vi "NMR T2 CPMG Sequence - Large Magnet - PN HPA - 2nd Setup.vi"() -> ()   [LabVIEW 2024]
uses:
  <instrlib>/niFgen/niFgen.llb/niFgen Output Mode.ctl
  <instrlib>/niFgen/niFgen.llb/niFgen Waveform Type.ctl
  <instrlib>/niFgen/niFgen.llb/niFgen_ctl Trigger DigEdge - Edge Values (Ring).ctl
  <instrlib>/niFgen/niFgen.llb/niFgen_ctl Trigger Source Values (Ring).ctl
  <instrlib>/niFgen/niFgen.llb/niFgen Trigger Mode.ctl
  <instrlib>/niScope/Controls/niScope acquisition type.ctl
  <instrlib>/niScope/Controls/niScope trigger slope.ctl
  <instrlib>/niScope/Controls/niScope trigger source.ctl
  <vilib>/Analysis/2dsp.llb/Integral Method.ctl
  <vilib>/Analysis/8numeric.llb/1D Numeric Integration.vi
  <vilib>/Utility/file.llb/Read Delimited Spreadsheet (DBL).vi
  <instrlib>/niFgen/niFgen.llb/niFgen Create Waveform (DBL).vi
  <instrlib>/niScope/Configure/Trigger/niScope Configure Trigger Edge.vi
  <instrlib>/niFgen/niFgen.llb/niFgen Configure Digital Edge Start Trigger.vi
  <instrlib>/niScope/Acquire/Fetch/niScope Fetch Cluster.vi
  <vilib>/Waveform/WDTFileIO.llb/Export Waveform To Spreadsheet File.vi
  <vilib>/Analysis/NI_AALPro.lvlib
panel:
  out "Pulse Echos - Current Scan":waveform(dbl)(graph)={"t0"=timestamp(0 s since 1904-01-01), "dt"=0.0012610340479192938, "Y"=array[3965 elements]} caption="Waveform Graph"
  in  "Write Output to File?":bool=TRUE
  out "Averaged T2 Decay":waveform(dbl)(graph)={"t0"=timestamp(0 s since 1904-01-01), "dt"=0.0012610340479192938, "Y"=array[3965 elements]} caption="Waveform Graph"
  out "Scan Number":i32=8
  out "Signal Intensity (Integral)":dbl=0.6544283602926818 format="%0.4f"
  out "Extracted T2 Decay - Current Scan":waveform(dbl)(graph)={"t0"=timestamp(0 s since 1904-01-01), "dt"=0.0012610340479192938, "Y"=array[3965 elements]} caption="Waveform Graph"
  in  "Pulse Train File":path=path "C:/Users/MK92/OneDrive - University of South Carolina/Github Repos/Compact-NMR/System_development/Van-Hove/LabVIEW/7 us 90 Degree - 1.25 ms Tau - 1977 Pulses.txt"
  in  "Larmor Frequency":dbl=27410000.0 caption="Frequency" format="%.4p"
  in  "Number of Scans":i32=8
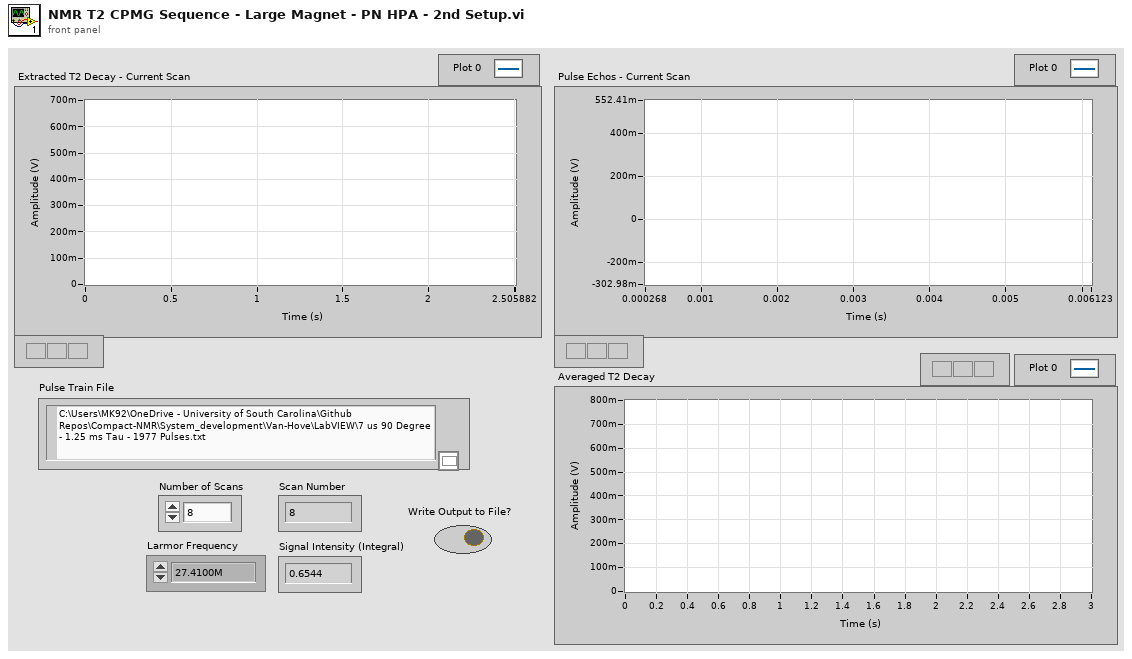
[diagram p1: front panel]
types:
  T1 = typedef "niFgen Output Mode.ctl" = u32
  T2 = typedef "niScope trigger source.ctl" = string
  T3 = typedef "niFgen_ctl Trigger Source Values (Ring).ctl" = string
  T4 = typedef "NI_AALPro.lvlib/Integral Method.ctl" = i32
  T5 = typedef "niScope trigger slope.ctl" = i32
  T6 = typedef "niScope acquisition type.ctl" = i32
  T7 = typedef "niFgen Trigger Mode.ctl" = i32
  T8 = typedef "niFgen_ctl Trigger DigEdge - Edge Values (Ring).ctl" = i32
  T9 = typedef "niFgen Waveform Type.ctl" = i32
  T10 = cluster{"relativeInitialX":dbl, "xIncrement":dbl, "wfm":dbl[]}
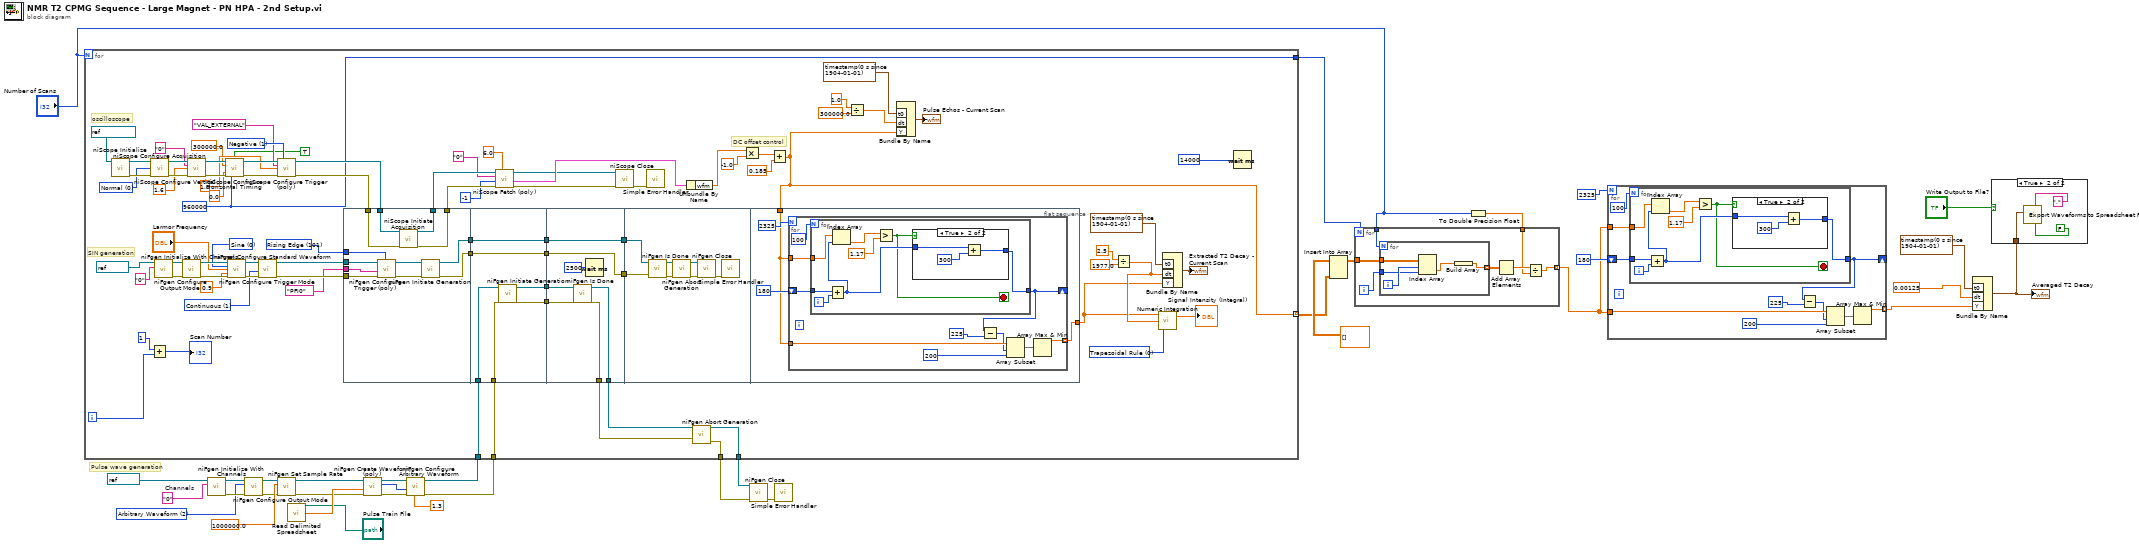
[diagram p0: block diagram]
diagram:
  w21 = "0"  # Channels
  w20 = T1 2 items=["Standard Function", "Frequency List", "Arbitrary Waveform", "Arbitrary Sequence", "Script"] ("output mode")
  # "Pulse wave generation"
  n1 = call <instrlib>:"niFgen Initialize With Channels.vi"("Channel Name"=w21, "Resource Name"=refnum<k15> "Dev1" ("FGEN Resource Name 2")) -> ("error out"=w24:errorcluster, "Instrument Handle Out"=w25:refnum<k15>)  [unwired: 8 in]
  n2 = call <instrlib>:"niFgen Configure Output Mode.vi"("error in (no error)"=w24, "Output Mode (default: 0=Standard Function)"=w20, "Instrument Handle"=w25) -> ("error out"=w28:errorcluster, "Instrument Handle Out"=w27:refnum<k15>)  [unwired: 6 in]
  n3 = call <instrlib>:"niFgen Set Sample Rate.vi"("error in (no error)"=w28, "Sample Rate (Samp/s)"=1000000.0 ("Sample Rate"), "Instrument Handle"=w27) -> ("error out"=w31:errorcluster, "Instrument Handle Out"=w30:refnum<k15>)  [unwired: 7 in]
  n4 = call-poly <vilib>:"Read Delimited Spreadsheet.vi"("file path (dialog if empty)"="Pulse Train File") -> ("first row"=w32:dbl[])  [unwired: 9 in, 5 out]
  n5 = call-poly <instrlib>:"niFgen Create Waveform (poly).vi"("error in (no error)"=w31, "Waveform Data Array"=w32, "Instrument Handle"=w30) -> ("error out"=w34:errorcluster, "Waveform Handle"=w35:i32, "Instrument Handle Out"=w33:refnum<k15>)  [unwired: 6 in]
  n6 = call <instrlib>:"niFgen Configure Arbitrary Waveform.vi"("Gain"=1.3, "error in (no error)"=w34, "Waveform Handle"=w35, "Instrument Handle"=w33) -> ("error out"=w19:errorcluster, "Instrument Handle Out"=w18:refnum<k15>)  [unwired: 6 in]
  n7 = for {
    N: "Number of Scans" -> [_]
    tunnel: w19 -> [w99]
    tunnel: w18 -> [w98]
    tunnel: [w97] -> w16
    tunnel: [w96] -> w15
    tunnel: [w36] -> w12 mode=indexing
    tunnel: [w47] -> w9
    i -> [w54]
    w56 = T4 0 items=["Trapezoidal Rule", "Simpson's Rule", "Simpson's 3/8 Rule", "Bode Rule"] ("integration method")
    w47 = 960000 ("min record length")
    w84 = T5 1 items=["Positive", "Negative"] ("trigger slope")
    w85 = T6 0 items=["Normal"=0, "Flex Res"=1, "DDC"=3] ("acquisition Type")
    w104 = T7 1 items=["Single", "Continuous", "Stepped", "Burst"] ("Trigger Mode (default: 1=continuous)")
    w108 = T8 101 items=["Rising Edge"=101, "Falling Edge"=102] ("Edge (Rising)")
    w109 = T9 0 items=["Sine", "Square", "Triangle", "Ramp Up", "Ramp Down", "DC", "Noise", "User"] ("Waveform")
    # "SIN generation"
    # "oscilloscope"
    # "DC offset control"
    n8 = call <instrlib>:"niScope Initialize.vi"("resource name"=refnum<k15> "PXI1Slot4") -> ("instrument handle"=w86:refnum<k15>, "error out"=w87:errorcluster)  [unwired: 13 in]
    n9 = call <instrlib>:"niScope Configure Acquisition.vi"("instrument handle"=w86, "acquisition Type"=w85, "error in"=w87) -> ("instrument handle out"=w89:refnum<k15>, "error out"=w90:errorcluster)  [unwired: 11 in]
    n10 = Add(x=1, y=w54) -> (x+y=→"Scan Number":i32)
    n11 = call <instrlib>:"niFgen Initialize With Channels.vi"("Channel Name"="0", "Resource Name"=refnum<k15> "Dev2" ("Sine Wave Module")) -> ("error out"=w114:errorcluster, "Instrument Handle Out"=w117:refnum<k15>)  [unwired: 8 in]
    n12 = call <instrlib>:"niFgen Configure Output Mode.vi"("error in (no error)"=w114, "Instrument Handle"=w117) -> ("error out"=w113:errorcluster, "Instrument Handle Out"=w116:refnum<k15>)  [unwired: 7 in]
    n13 = call <instrlib>:"niScope Configure Vertical.vi"("instrument handle"=w89, "channels"="0", "vertical range"=1.6, "error in"=w90) -> ("instrument handle out"=w91:refnum<k15>, "error out"=w92:errorcluster)  [unwired: 10 in]
    n14 = call <instrlib>:"niScope Configure Horizontal Timing.vi"("instrument handle"=w91, "enforce realtime"=TRUE, "min sample rate"=300000.0, "reference position"=0.0, "error in"=w92, "min record length"=w47) -> ("instrument handle out"=w93:refnum<k15>, "error out"=w94:errorcluster)  [unwired: 8 in]
    n15 = call <instrlib>:"niFgen Configure Standard Waveform.vi"("Instrument Handle"=w116, "Waveform"=w109, "Frequency"="Larmor Frequency", "Amplitude"=0.9, "error in (no error)"=w113) -> ("Instrument Handle Out"=w115:refnum<k15>, "error out"=w112:errorcluster)  [unwired: 9 in]
    n16 = call <instrlib>:"niFgen Configure Trigger Mode.vi"("error in (no error)"=w112, "Trigger Mode (default: 1=continuous)"=w104, "Instrument Handle"=w115) -> ("error out"=w107:errorcluster, "Instrument Handle Out"=w105:refnum<k15>)  [unwired: 7 in]
    n17 = call-poly <instrlib>:"niScope Configure Trigger (poly).vi"("instrument handle"=w93, "trigger slope"=w84, "trigger source"=T2 "VAL_EXTERNAL", "trigger level"=1.0, "error in"=w94) -> ("instrument handle out"=w78:refnum<k15>, "error out"=w77:errorcluster)  [unwired: 9 in]
    n18 = flat-sequence {
      tunnel: w108 -> [w128]
      tunnel: w107 -> [w127]
      tunnel: T3 "PFI0" ("Source") -> [w126]
      tunnel: w105 -> [w125]
      tunnel: w78 -> [w123]
      tunnel: w77 -> [w122]
      tunnel: [w121] -> w76
      tunnel: [w120] -> w75
      tunnel: [w119] -> w65
      tunnel: [w118] -> w62
      tunnel: w99 -> [w135]
      tunnel: w98 -> [w134]
      tunnel: [w133] -> w69
      tunnel: [w132] -> w68
      tunnel: [w131] -> w66
      tunnel: w65 -> [w131]
      tunnel: [w130] -> w63
      tunnel: w62 -> [w130]
      tunnel: [w141] -> w102
      tunnel: [w140] -> w101
      tunnel: w69 -> [w139]
      tunnel: w68 -> [w138]
      tunnel: [w137] -> w67
      tunnel: w66 -> [w137]
      tunnel: [w136] -> w64
      tunnel: w63 -> [w136]
      tunnel: w67 -> [w144]
      tunnel: w64 -> [w143]
      tunnel: w36 -> [w150]
      tunnel: [w152] -> w46
      frame #0 {
        n19 = call-poly <instrlib>:"niFgen Configure Trigger (poly).vi"("Edge (Rising)"=w128, "error in (no error)"=w127, "Source"=w126, "Instrument Handle"=w125) -> ("error out"=w124:errorcluster, "Instrument Handle Out"=w129:refnum<k15>)  [unwired: 6 in]
        n20 = call <instrlib>:"niScope Initiate Acquisition.vi"("instrument handle"=w123, "error in"=w122) -> ("instrument handle out"=w121:refnum<k15>, "error out"=w120:errorcluster)  [unwired: 12 in]
        n21 = call <instrlib>:"niFgen Initiate Generation.vi"("error in (no error)"=w124, "Instrument Handle"=w129) -> ("error out"=w118:errorcluster, "Instrument Handle Out"=w119:refnum<k15>)  [unwired: 8 in]
      }
      frame #1 {
        n22 = call <instrlib>:"niFgen Initiate Generation.vi"("error in (no error)"=w135, "Instrument Handle"=w134) -> ("error out"=w132:errorcluster, "Instrument Handle Out"=w133:refnum<k15>)  [unwired: 8 in]
      }
      frame #2 {
        n23 = call <instrlib>:"niFgen Is Done.vi"("error in (no error)"=w138, "Instrument Handle"=w139) -> ("error out"=w141:errorcluster, "Instrument Handle Out"=w140:refnum<k15>)  [unwired: 7 in, 1 out]
        n24 = Wait (ms)(milliseconds to wait=u32 2500) -> ()  [unwired: 1 out]
      }
      frame #3 {
        n25 = call <instrlib>:"niFgen Is Done.vi"("error in (no error)"=w143, "Instrument Handle"=w144) -> ("error out"=w147:errorcluster, "Instrument Handle Out"=w146:refnum<k15>)  [unwired: 7 in, 1 out]
        n26 = call <instrlib>:"niFgen Abort Generation.vi"("error in (no error)"=w147, "Instrument Handle"=w146) -> ("error out"=w148:errorcluster, "Instrument Handle Out"=w149:refnum<k15>)  [unwired: 8 in]
        n27 = call <instrlib>:"niFgen Close.vi"("error in (no error)"=w148, "Instrument Handle"=w149) -> ("error out"=w145:errorcluster)  [unwired: 9 in]
        n28 = call <vilib>:"Simple Error Handler.vi"("error in (no error)"=w145) -> ()  [unwired: 4 in, 5 out]
      }
      frame #4 {
        n29 = for {
          N: 2325 -> [_]
          tunnel: [w162] -> w152 mode=indexing
          tunnel: w150 -> [w161]
          shift-right: [w156] -> _
          shift-left: 180 -> [w157]
          tunnel: w150 -> [w155]
          n30 = for {
            N: 100 -> [_]
            tunnel: w155 -> [w167]
            tunnel: w157 -> [w170]
            tunnel: [w165] -> w156
            i -> [w171]
            stop <- w164 stop-if-true
            n31 = Add(x=w170, y=w171) -> (x+y=w166:i32)
            n32 = Index Array(array=w167, index=w166) -> (element=w168:dbl)
            n33 = Greater?(x=w168, y=1.17) -> (0:w164:bool)
            n34 = case shown="True" w164 {
              tunnel: w166 -> [w172 w173]
              tunnel: [w172 w175] -> w165
              frame False {
              }
              frame True {
                n35 = Add(x=w173, y=300) -> (x+y=w175:i32)
              }
            }
          }
          n36 = Subtract(x=w156, y=225) -> (x-y=w158:i32)
          n37 = Array Subset(array=w161, index=w158, length=200 ("y")) -> (w163:dbl[])
          n38 = Array Max & Min(array=w163) -> (max value=w162:dbl)  [unwired: 3 out]
        }
      }
    }
    n39 = call-poly <instrlib>:"niScope Fetch (poly).vi"("timeout"=6.0, "error in"=w75, "numSamples"=-1, "channels"="0", "instrument handle"=w76) -> ("error out"=w48:errorcluster, "waveform"=w51:T10, "instrument handle out"=w49:refnum<k15>)  [unwired: 3 in, 1 out]
    n40 = call <instrlib>:"niScope Close.vi"("instrument handle"=w49, "error in"=w48) -> ("error out"=w95:errorcluster)  [unwired: 13 in]
    n41 = call <vilib>:"Simple Error Handler.vi"("error in (no error)"=w95) -> ()  [unwired: 4 in, 5 out]
    n42 = Unbundle By Name(w51) -> ("wfm"=w40:dbl[])
    n43 = call <instrlib>:"niFgen Abort Generation.vi"("error in (no error)"=w102, "Instrument Handle"=w101) -> ("error out"=w97:errorcluster, "Instrument Handle Out"=w96:refnum<k15>)  [unwired: 8 in]
    n44 = Multiply(x=w40, y=-1.0) -> (x*y=w37:dbl[])
    n45 = Add(x=w37, y=0.185) -> (x+y=w36:dbl[])
    n46 = Divide(x=1.0, y=300000.0) -> (x/y=w41:dbl)
    n47 = Bundle By Name("t0"=timestamp(0 s since 1904-01-01), "dt"=w41, "Y"=w36) -> (→"Pulse Echos - Current Scan":waveform(dbl))  [unwired: 1 in]
    n48 = Divide(x=2.5, y=1977.0) -> (x/y=w57:dbl)
    n49 = call-poly <vilib>:"Numeric Integration.vi"("integration method"=w56, "dt"=w57, "Input Array"=w46) -> ("result"=→"Signal Intensity (Integral)":dbl)  [unwired: 1 out]
    n50 = Bundle By Name("t0"=timestamp(0 s since 1904-01-01), "dt"=w57, "Y"=w46) -> (→"Extracted T2 Decay - Current Scan":waveform(dbl))  [unwired: 1 in]
    n51 = Wait (ms)(milliseconds to wait=u32 14000 ("Delay Time (ms)")) -> ()  [unwired: 1 out]
  }
  n52 = call <instrlib>:"niFgen Close.vi"("error in (no error)"=w16, "Instrument Handle"=w15) -> ("error out"=w17:errorcluster)  [unwired: 9 in]
  n53 = call <vilib>:"Simple Error Handler.vi"("error in (no error)"=w17) -> ()  [unwired: 4 in, 5 out]
  n54 = Insert Into Array(array=dbl[][] [], new element=w12) -> (w14:dbl[][])  [unwired: 2 in]
  n55 = To Double Precision Float(number="Number of Scans") -> (double precision float=w11:dbl)
  n56 = for {
    N: w9 -> [_]
    tunnel: w14 -> [w182]
    tunnel: [w178] -> w5 mode=indexing
    tunnel: "Number of Scans" -> [w177]
    tunnel: w11 -> [w176]
    i -> [w181]
    n57 = for {
      N: w177 -> [_]
      tunnel: w182 -> [w187]
      tunnel: w181 -> [w185]
      tunnel: [w183] -> w180 mode=indexing
      i -> [w186]
      n58 = Index Array(array=w187, index (row)=w186, index (col)=w185) -> (element=w184:dbl)
      n59 = Build Array(w184) -> (w183:dbl[])
    }
    n60 = Add Array Elements(numeric array=w180) -> (sum=w179:dbl)
    n61 = Divide(x=w179, y=w176) -> (x/y=w178:dbl)
  }
  n62 = for {
    N: 2325 -> [_]
    tunnel: [w196] -> w4 mode=indexing
    tunnel: w5 -> [w195]
    shift-right: [w190] -> _
    shift-left: 180 -> [w191]
    tunnel: w5 -> [w189]
    n63 = for {
      N: 100 -> [_]
      tunnel: w189 -> [w201]
      tunnel: w191 -> [w204]
      tunnel: [w199] -> w190
      i -> [w205]
      stop <- w198 stop-if-true
      n64 = Add(x=w204, y=w205) -> (x+y=w200:i32)
      n65 = Index Array(array=w201, index=w200) -> (element=w202:dbl)
      n66 = Greater?(x=w202, y=1.17) -> (0:w198:bool)
      n67 = case shown="True" w198 {
        tunnel: w200 -> [w206 w207]
        tunnel: [w206 w209] -> w199
        frame False {
        }
        frame True {
          n68 = Add(x=w207, y=300) -> (x+y=w209:i32)
        }
      }
    }
    n69 = Subtract(x=w190, y=225) -> (x-y=w192:i32)
    n70 = Array Subset(array=w195, index=w192, length=200 ("y")) -> (w197:dbl[])
    n71 = Array Max & Min(array=w197) -> (max value=w196:dbl)  [unwired: 3 out]
  }
  n72 = Bundle By Name("t0"=timestamp(0 s since 1904-01-01), "dt"=0.00125 ("y"), "Y"=w4) -> (w2:waveform(dbl))  [unwired: 1 in]
  "Averaged T2 Decay" <- w2
  n73 = case shown="True" "Write Output to File?" {
    tunnel: w2 -> [_ w210]
    frame False {
    }
    frame True {
      n74 = call-poly <vilib>:"Export Waveforms to Spreadsheet File.vi"("header? (write header:T)"=FALSE, "delimiter (Tab)"=",", "waveform"=w210) -> ()  [unwired: 7 in, 2 out]
    }
  }
